vi "DashboardShutdown.vi"(8 "Dashboard":refnum<k24>, 11 "error in":errorcluster) -> (0 "Response":cluster{"Message":string, "Succeed":bool}, 3 "error out":errorcluster)   [LabVIEW 2023, in "UnderAutomation.UniversalRobots.lvlib"]
uses:
  UnderAutomation.UniversalRobots.lvlib
  C:/Users/fg/Documents/UniversalRobots.vi/UnderAutomation.UniversalRobots/lib/UnderAutomation.UniversalRobots.dll
  lib/UnderAutomation.UniversalRobots.dll
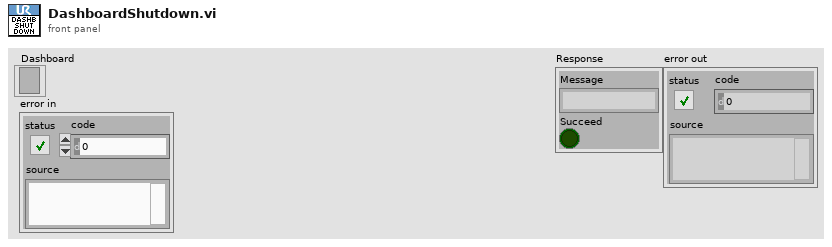
[diagram p1: front panel]
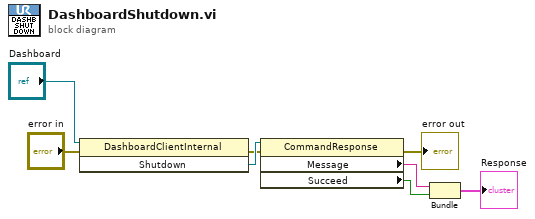
[diagram p0: block diagram]
diagram:
  n1 = invoke class="DashboardClientInternal" method="Shutdown"(reference="Dashboard", error in="error in") -> (error out=w2:errorcluster, "Shutdown"=w7:refnum<k24>)  [unwired: 1 in, 1 out]
  n2 = property class="CommandResponse"(reference=w7, error in=w2) -> (error out=→"error out":errorcluster, "Message"=w6:string, "Succeed"=w5:bool)  [unwired: 1 out]
  n3 = Bundle("Message"=w6, "Succeed"=w5) -> (→"Response":cluster{"Message":string, "Succeed":bool})  [unwired: 1 in]
